vi "SMTP Email Send Data Attachment.vi"(0 "smtp session":T1, 1 "character set":string, 5 "data":string, 11 "error in (no error)":errorcluster, 12 "binary (F)":bool, 14 "translit":string) -> (4 "smtp session out":T1, 15 "error out":errorcluster)   [LabVIEW 2012, in "NewNI_SMTPEmail.lvlib"]
uses:
  NewNI_SMTPEmail.lvlib
  SMTP Email Session.ctl
panel:
  in  "buffered tcp connection":refnum<k5>
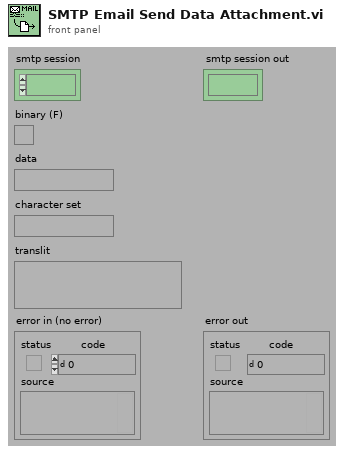
[diagram p1: front panel]
types:
  T1 = typedef "NewNI_SMTPEmail.lvlib/SMTP Email Session.ctl" = refnum<k1>
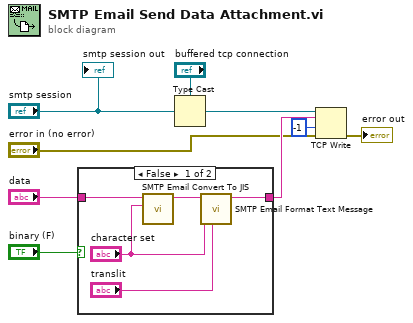
[diagram p0: block diagram]
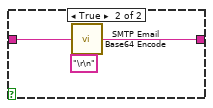
[diagram p2: hidden frame]
diagram:
  n1 = case shown="False" "binary (F)" {
    tunnel: [w14 w16] -> w6
    tunnel: "data" -> [w11 w17]
    frame False {
      n2 = call "SMTP Email Convert To JIS.vi"("character set"="character set", "text in"=w11) -> ("text out"=w10:string)  [unwired: 9 out]
      n3 = call "SMTP Email Format Text Message.vi"("translit"="translit", "character set"="character set", "text"=w10) -> ("formated text"=w14:string)  [unwired: 2 in, 4 out]
    }
    frame True {
      n4 = call "SMTP Email Base64 Encode.vi"("Normal String"=w17, "Line separator (\\n)"="\r\n") -> ("Base64 String"=w16:string)
    }
  }
  n5 = Type Cast(type="buffered tcp connection", x="smtp session") -> (*(type *) &x=w3:refnum<k5>)
  n6 = TCP Write(connection ID=w3, data in=w6, error in (no error)="error in (no error)", 9:-1 ("timeout ms (25000)")) -> (error out=→"error out":errorcluster)  [unwired: 2 out]
  "smtp session out" <- "smtp session"
